vi "Write trackID.vi"(8 "error in (no error)":errorcluster, 10 "trackID":dbl, 11 "NewScienceTarget in":refnum<class "NewScienceTarget.lvclass">) -> (0 "error out":errorcluster, 3 "NewScienceTarget out":refnum<class "NewScienceTarget.lvclass">)   [LabVIEW 2014, in "TCSDataDefinitions.lvlib" / "TCSPublicStatus.lvlib" / "NewScienceTarget.lvclass"]
uses:
  NewScienceTarget.lvclass
  NewScienceTarget.lvclass/NewScienceTarget.ctl
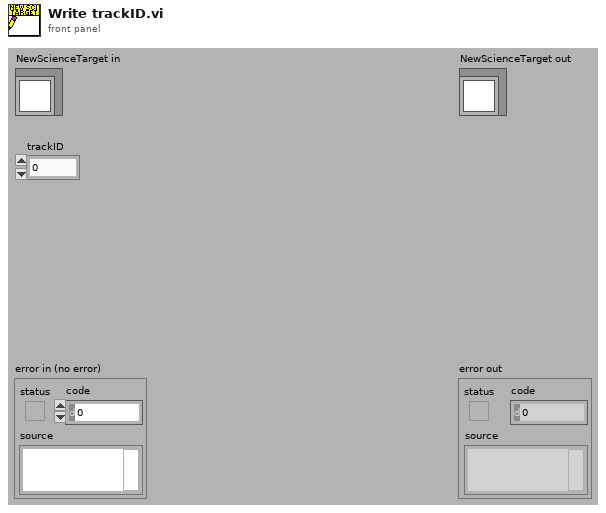
[diagram p1: front panel]
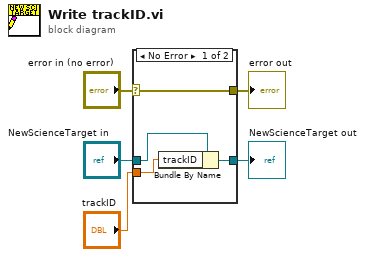
[diagram p0: block diagram]
diagram:
  n1 = case shown="No Error" "error in (no error)" {
    selector: "error in (no error)" -> [w9 w10]
    tunnel: [w9 w10] -> w4
    tunnel: [w7 w11] -> w2
    tunnel: "NewScienceTarget in" -> [w8 w11]
    tunnel: "trackID" -> [w6 _]
    frame No Error {
      n2 = Bundle By Name(cluster=w8, "trackID"=w6) -> (w7:refnum<class "NewScienceTarget.lvclass">)
    }
    frame Error {
    }
  }
  "error out" <- w4
  "NewScienceTarget out" <- w2
